vi "MathCad cmd v2.vi"(3 "Slide Refnum":refnum<vi>, 4 "Arr Refnum":refnum<vi>, 5 "MathCAD variables":T1, 6 "MathCAD cmds":T2, 7 "Str Refnum":refnum<vi>, 8 "error in":errorcluster, 9 "Clust Refnum":refnum<vi>, 10 "Num Refnum":refnum<vi>) -> (0 "first error out":errorcluster, 1 "errors":errorcluster[](array[cluster]))   [LabVIEW 2015]
uses:
  mathcad/Simple/MathCAD cmd.ctl
  MathCAD results ref.ctl
panel:
  in  "Mathcad.IMathcadApplication":refnum<k7>
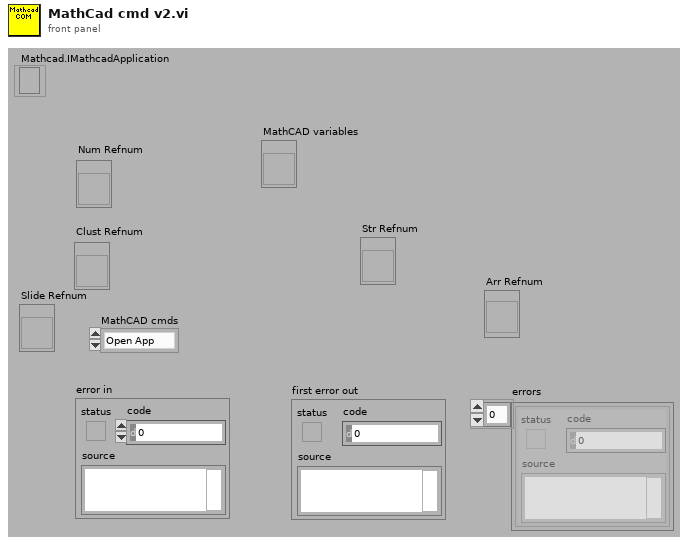
[diagram p1: front panel]
types:
  T1 = typedef "MathCAD results ref.ctl" = refnum<vi>
  T2 = typedef "MathCAD cmd.ctl" = enum16{"Open App", "Open Worksheet", "Close Worksheet", "Load Variable Ref", "Send Number", "Send Cluster", "Send Array", "Send String", "Calculate", "Get MathCAD data", "Close MathCAD"}
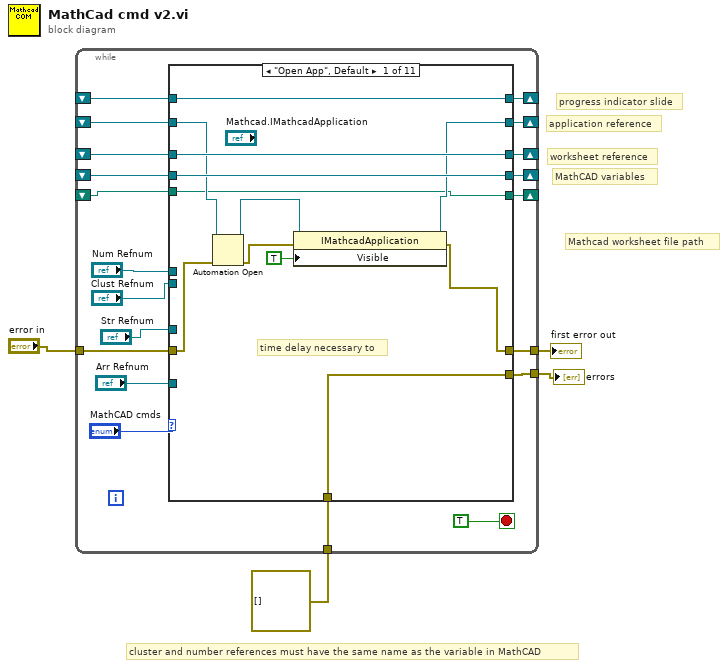
[diagram p0: block diagram]
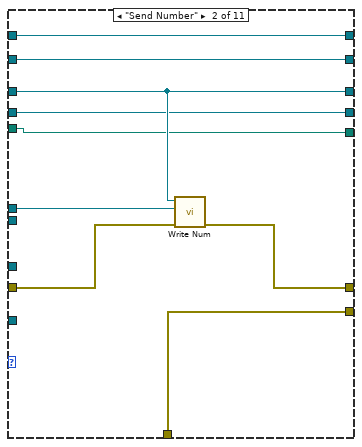
[diagram p2: hidden frame]
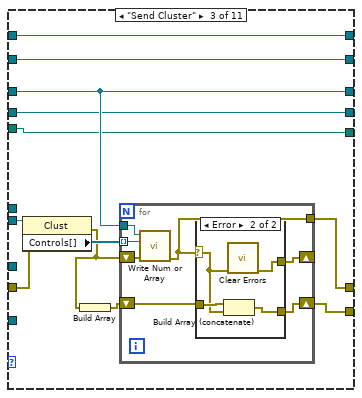
[diagram p3: hidden frame]
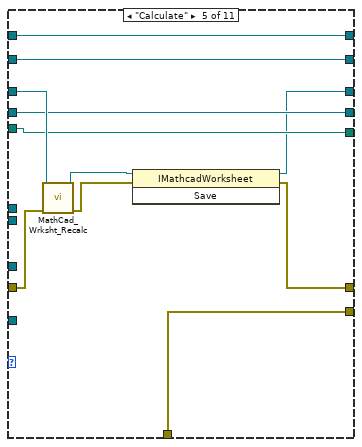
[diagram p6: hidden frame]
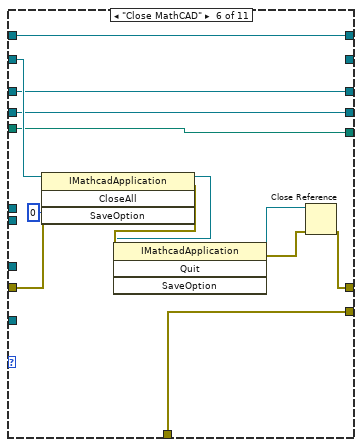
[diagram p7: hidden frame]
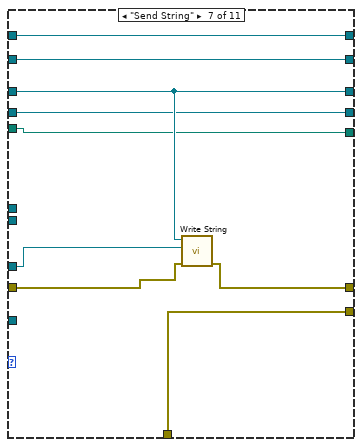
[diagram p8: hidden frame]
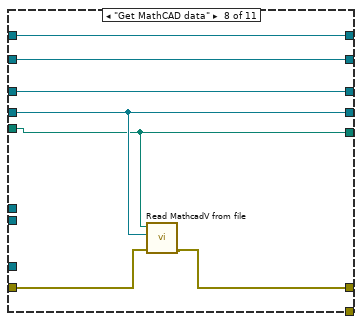
[diagram p9: hidden frame]
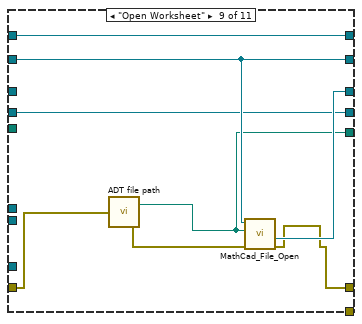
[diagram p10: hidden frame]
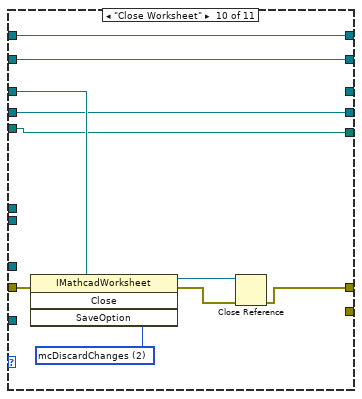
[diagram p11: hidden frame]
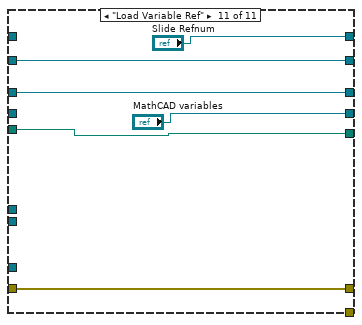
[diagram p12: hidden frame]
diagram:
  # "Mathcad worksheet file path"
  # "MathCAD variables"
  # "progress indicator slide"
  # "application reference"
  # "worksheet reference"
  # "cluster and number references must have the same name as the variable in MathCAD"
  n1 = while {
    shift-right: [w20] -> _
    shift-left: _ -> [w18]
    shift-right: [w19] -> _
    shift-left: _ -> [w17]
    tunnel: "error in" -> [w21]
    tunnel: [w22] -> w3
    tunnel: [w12] -> w2
    tunnel: errorcluster[] [] -> [w11]
    shift-right: [w10] -> _
    shift-left: _ -> [w9]
    shift-right: [w8] -> _
    shift-left: _ -> [w7]
    shift-right: [w6] -> _
    shift-left: _ -> [w5]
    stop <- TRUE stop-if-true
    n2 = case shown="\"Open App\", Default" "MathCAD cmds" {
      tunnel: [w28 w42 w54 w75 w78 w95 w108 w113 w119 w127 w138] -> w22
      tunnel: w21 -> [w27 w44 w52 w75 w86 w100 w109 w114 w122 w135 w138]
      tunnel: [w29 w45 w56 w77 w88 _ w110 w117 w124 w131 w139] -> w20
      tunnel: [w35 w43 w55 w76 w80 w99 w106 w116 w123 _ w140] -> w19
      tunnel: w18 -> [w32 w45 w56 w77 w88 w101 w110 w117 w124 w131 w139]
      tunnel: w17 -> [w35 w43 w55 w76 w87 w99 w106 w116 _ w133 w140]
      tunnel: "Num Refnum" -> [_ w41 _ _ _ _ _ _ _ _ _]
      tunnel: "Clust Refnum" -> [_ _ w53 _ _ _ _ _ _ _ _]
      tunnel: "Str Refnum" -> [_ _ _ _ _ _ w107 _ _ _ _]
      tunnel: "Arr Refnum" -> [_ _ _ _ _ _ _ _ _ _ _]
      tunnel: [w36 w40 w49 w74 w85 w98 w105 _ _ _ _] -> w12
      tunnel: w11 -> [w36 w40 _ w74 w85 w98 w105 _ _ _ _]
      tunnel: [w33 w39 w48 w73 w84 w97 w104 w115 w125 w132 "Slide Refnum"] -> w10
      tunnel: w9 -> [w33 w39 w48 w73 w84 w97 w104 w115 w125 w132 _]
      tunnel: w7 -> [w34 w38 w47 w72 w83 w96 w103 w112 w120 w130 _]
      tunnel: [w34 w38 w47 w72 w83 w96 w103 w112 w120 w130 "MathCAD variables"] -> w8
      tunnel: [w25 w37 w46 w71 w82 w89 w102 w111 w118 w126 w136] -> w6
      tunnel: w5 -> [w25 w37 w46 w71 w82 w89 w102 w111 _ w126 w136]
      frame "Open App", Default {
        # "time delay necessary to"
        n3 = Automation Open(error in (no error)=w27, Automation Refnum=w32) -> (Automation Refnum=w31:refnum<k7>, error out=w30:errorcluster)  [unwired: 2 in]
        n4 = property class="IMathcadApplication"(reference=w31, error in=w30, "Visible"=TRUE) -> (reference out=w29:refnum<k7>, error out=w28:errorcluster)
      }
      frame "Send Number" {
        n5 = call "Write Num.vi"("error in (no error)"=w44, "Ctl Refnum"=w41, "Worksheet Reference"=w43) -> ("error out"=w42:errorcluster)  [unwired: 8 in]
      }
      frame "Send Cluster" {
        n6 = property class="Clust"(reference=w53, error in=w52) -> (error out=w51:errorcluster, "Controls[]"=w57:refnum<vi>[])  [unwired: 1 out]
        n7 = Build Array(w51) -> (w50:errorcluster[])
        n8 = for {
          tunnel: w57 -> [w60] mode=indexing
          tunnel: w55 -> [w59]
          tunnel: [w58] -> w54
          shift-right: [w62] -> _
          shift-left: w51 -> [w61]
          shift-right: [w63] -> w49
          shift-left: w50 -> [w64]
          n9 = call "Write Num or Array.vi"("error in (no error)"=w61, "Ctl Refnum"=w60, "Worksheet Reference"=w59) -> ("error out"=w58:errorcluster)  [unwired: 8 in]
          n10 = case shown="Error" w58 {
            selector: w58 -> [w65 w68]
            tunnel: w64 -> [w66 w70]
            tunnel: [w66 w69] -> w63
            tunnel: [w65 w67] -> w62
            frame No Error {
            }
            frame Error {
              n11 = Build Array (concatenate)(w70, w68) -> (w69:errorcluster[])
              n12 = call <vilib>:"Clear Errors.vi"("error in (no error)"=w68) -> ("error out"=w67:errorcluster)  [unwired: 5 in, 1 out]
            }
          }
        }
      }
      frame "Send Array" {
      }
      frame "Calculate" {
        n13 = call "MathCad_Wrksht_Recalc.vi"("error in (no error)"=w86, "Worksheet Reference"=w87) -> ("error out"=w79:errorcluster, "Worksheet Reference"=w81:refnum<k7>)  [unwired: 8 in]
        n14 = invoke class="IMathcadWorksheet" method="Save"(reference=w81, error in=w79) -> (reference out=w80:refnum<k7>, error out=w78:errorcluster)  [unwired: 1 in, 1 out]
      }
      frame "Close MathCAD" {
        n15 = invoke class="IMathcadApplication" method="CloseAll"(reference=w101, error in=w100, "SaveOption"=0) -> (reference out=w93:refnum<k7>, error out=w94:errorcluster)  [unwired: 1 in, 2 out]
        n16 = invoke class="IMathcadApplication" method="Quit"(reference=w93, error in=w94) -> (reference out=w92:refnum<k7>, error out=w91:errorcluster)  [unwired: 2 in, 2 out]
        n17 = Close Reference(reference=w92, error in (no error)=w91) -> (error out=w95:errorcluster)
      }
      frame "Send String" {
        n18 = call "Write String.vi"("error in (no error)"=w109, "Ctl Refnum"=w107, "Worksheet Reference"=w106) -> ("error out"=w108:errorcluster)  [unwired: 8 in]
      }
      frame "Get MathCAD data" {
        n19 = call "Read MathcadV from file.vi"("error in (no error)"=w114, "Ctl Refnum"=w112, "Path"=w111) -> ("error out"=w113:errorcluster)  [unwired: 8 in]
      }
      frame "Open Worksheet" {
        n20 = call "ADT file path.vi"("error in"=w122) -> ("error out"=w121:errorcluster, "dup path"=w118:path)
        n21 = call "MathCad_File_Open.vi"("error in (no error)"=w121, "Worksheet File"=w118, "Mathcad.IMathcadApplication"=w124) -> ("error out (no error)"=w119:errorcluster, "Worksheet Reference"=w123:refnum<k7>)  [unwired: 5 in, 2 out]
      }
      frame "Close Worksheet" {
        w134 = 2 items=["mcSaveChanges", "mcPromptToSaveChanges", "mcDiscardChanges"] ("SaveOption")
        n22 = invoke class="IMathcadWorksheet" method="Close"(reference=w133, error in=w135, "SaveOption"=w134) -> (reference out=w129:refnum<k7>, error out=w128:errorcluster)  [unwired: 1 in, 2 out]
        n23 = Close Reference(reference=w129, error in (no error)=w128) -> (error out=w127:errorcluster)
      }
      frame "Load Variable Ref" {
      }
    }
  }
  "first error out" <- w3
  "errors" <- w2
